vi "PH_AxisGUI_BaseClass.panel.vi"(0 "object ref":refnum<vi>, 5 "error in (no error)":errorcluster) -> (19 "error out":errorcluster)   [LabVIEW 2014, in "PH_AxisGUI_BaseClass.lvlib"]
doc: "License Agreement for this software:\n\nCopyright (C)\nGesellschaft für Schwerionenforschung, GSI\nPlanckstr. 1\n64291 Darmstadt\nGermany\n\nContact: D.Beck@gsi.de \n\nThis program is free software; you can redistribute it and/or modify it under the terms of the GNU General Public License as published by the Free Software Foundation; either version 2 of the license, or (at your option) any later version.\n\nThis program is distributed in the hope that it will be useful, but WITHOUT ANYW ARRANTY; without even the implied warranty of MERCHANTABILITY or FITNESS FOR A PARTICULAR PURPOSE. See the GNU General License for more details (http://www.gnu.org).\n\nGesellschaft für Schwerionenforschung, GSI\nPlanckstr. 1, 64291 Darmstadt, Germany\nFor all questions and ideas contact: M.Richter@gsi.de, H.Brand@gsi.de or D.Beck@gsi.de.\nLast update: 18-DEC-2002"
uses:
  PH_AxisGUI_BaseClass.lvlib
  PH_Stepmotor_BaseClass/PH_Stepmotor_BaseClass.Axis Settings.ctl
  PH_Stepmotor_BaseClass/PH_Stepmotor_BaseClass.Motor Type.ctl
  PH_Stepmotor_BaseClass/PH_Stepmotor_BaseClass.Axis Address.ctl
  PH_Stepmotor_BaseClass/PH_Stepmotor_BaseClass.Axis Activity.ctl
  PH_AxisGUI_BaseClass.Axis GUI Refs.ctl
  PH_Stepmotor_BaseClass/PH_Stepmotor_BaseClass.Axis Direction.ctl
  PH_Common/PH_Common.lvlib
  PH_Stepmotor_BaseClass/PH_Stepmotor_BaseClass.lvlib
  PH_Class/PH_Class.lvlib
panel:
  out "Activity":T1
  out "Status Bar":u32(colorbox)=16777088 caption="Axis1"
  out "Status":u32(colorbox)=6618880 caption="Axis1"
  in  "Stop":bool caption="SetZero"
  in  "Tab Control":enum32{"Move", "Settings", "Info"}(tab)
  in  "Clear Error":bool
  in  "Forth":bool caption="? Steps"
  in  "Back":bool caption="? Steps"
  in  "Target":string="0" caption="Steps"
  in  "Settings":T2={"Sign change"=FALSE, "Width"=0.0, "Calibration"=0.0, "Unit"="Steps", "Motor Type"=enum."Unspecific", "Unit Width"="", "Unit CF"=""}
  out "Address":T4={"Instance"="N/A", "Motor Nr"=0}
  in  "SetZero":bool
  in  "Reset":bool
  in  "Delete":bool
  # "PCS"
  # "3.40"
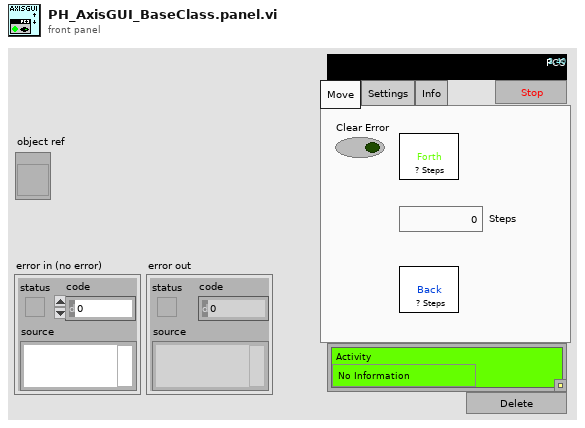
[diagram p1: front panel]
types:
  T1 = typedef "PH_Stepmotor_BaseClass.lvlib/PH_Stepmotor_BaseClass.Axis Activity.ctl" = enum16{"No Information", "stopped", "running", "Failure", "Alarm", "stopped at backward ES", "stopped at foreward ES"}
  T2 = typedef "PH_Stepmotor_BaseClass.lvlib/PH_Stepmotor_BaseClass.Axis Settings.ctl" = cluster{"Sign change":bool, "Width":dbl, "Calibration":dbl, "Unit":string, "Motor Type":T3, "Unit Width":string, "Unit CF":string}
  T3 = typedef "PH_Stepmotor_BaseClass.lvlib/PH_Stepmotor_BaseClass.Motor Type.ctl" = enum16{"Unspecific", "OWIS 49.120.2633", "OWIS 49.060.1033", "OWIS 43.040.2558", "Diamond Motion 2200 series", "OWIS 49.120.266B.MV6", "Calorimeter", "Linear Stage 1", "MICOS VT-80", "MICOS VT-80 S", "Standa Rotstage nt0.95A", "PUF RA 320.200", "PUF RA 800.200", "PUF RA 800.400", "PUF RA 400.50", "1324.nn.800.50", "1324.n9c.800.50", "1324.nn.320.200", "1324.nn.400.200", "1324.nn.800.200", "1324.nn.400.50", "1324.8c9c.800.50", "1324.8c9c.400.200"}
  T4 = typedef "PH_Stepmotor_BaseClass.lvlib/PH_Stepmotor_BaseClass.Axis Address.ctl" = cluster{"Instance":string, "Motor Nr":i32}
  T5 = typedef "PH_AxisGUI_BaseClass.lvlib/PH_AxisGUI_BaseClass.Axis GUI Refs.ctl" = cluster{"Back":refnum<vi>, "Forth":refnum<vi>, "Status":refnum<vi>, "Target":refnum<vi>, "Address":refnum<vi>, "Status Bar":refnum<vi>, "Settings":refnum<vi>, "Activity":refnum<vi>, "Clear Error":refnum<vi>}
  T6 = typedef "PH_Stepmotor_BaseClass.lvlib/PH_Stepmotor_BaseClass.Axis Direction.ctl" = enum16{"forward", "backward"}
  T7 = typedef "PH_AxisGUI_BaseClass.lvlib/PH_AxisGUI_BaseClass.i attribute.ctl" = cluster{"Axes":T8[]}
  T8 = typedef "PH_AxisGUI_BaseClass.lvlib/PH_AxisGUI_BaseClass.Axis Attributes.ctl" = cluster{"Axis GUI Refs":T5, "Address":T4, "Name":string, "Label \"Back\"":string, "Labell \"Forth\"":string, "Moving?":bool}
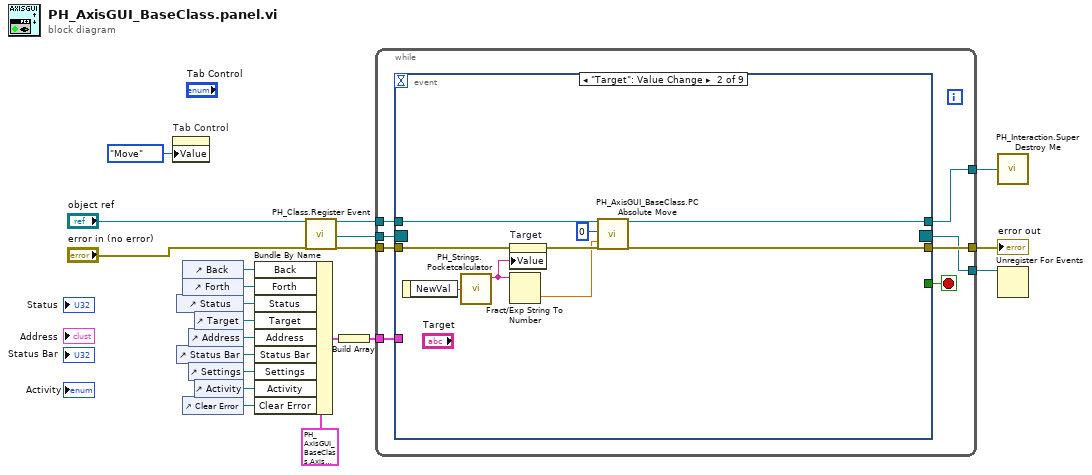
[diagram p0: block diagram]
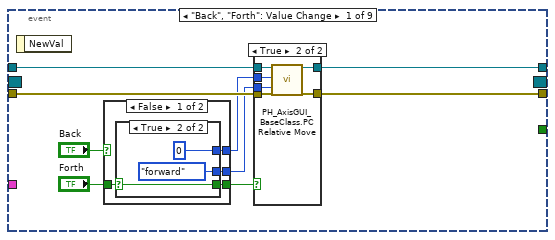
[diagram p2: hidden frame]
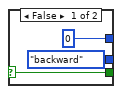
[diagram p3: hidden frame]
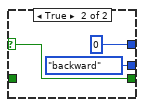
[diagram p4: hidden frame]
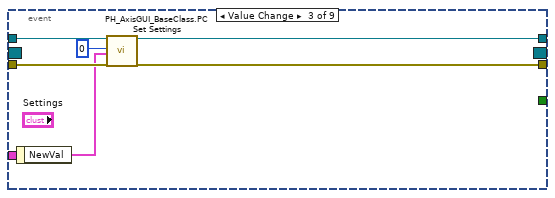
[diagram p6: hidden frame]
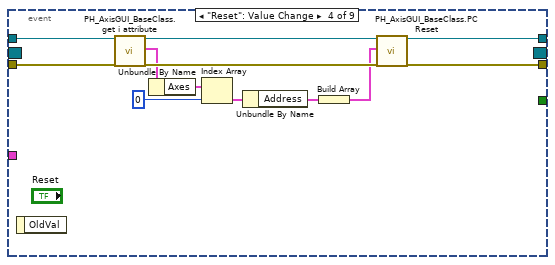
[diagram p7: hidden frame]
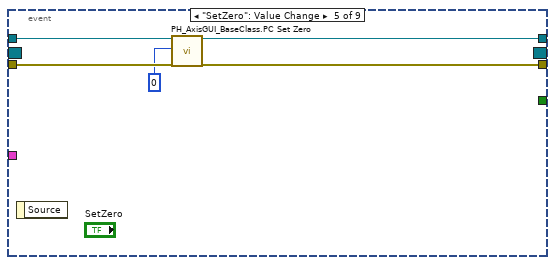
[diagram p8: hidden frame]
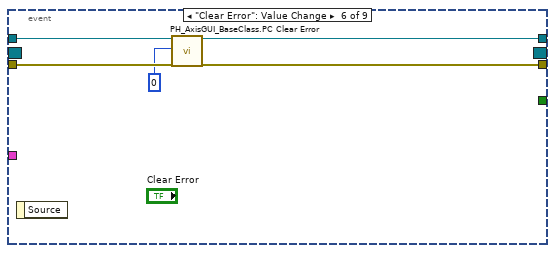
[diagram p9: hidden frame]
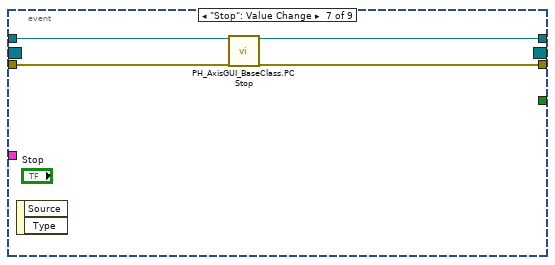
[diagram p10: hidden frame]
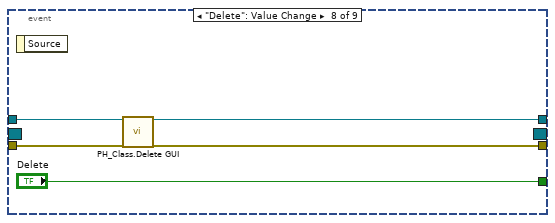
[diagram p11: hidden frame]
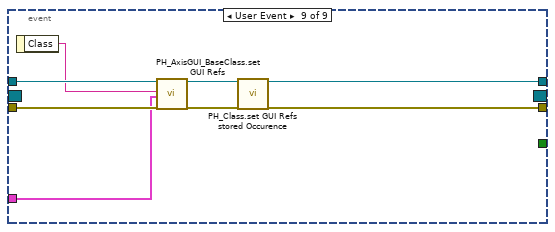
[diagram p12: hidden frame]
diagram:
  n1 = property on="Tab Control" class="TabCtl (strict)"("Value"=enum32{"Move", "Settings", "Info"}."Move" ("Tab Control")) -> ()  [unwired: 2 in, 2 out]
  n2 = control-ref of="Status"() -> (w15:refnum<vi>)
  n3 = control-ref of="Status Bar"() -> (w11:refnum<vi>)
  n4 = control-ref of="Back"() -> (w17:refnum<vi>)
  n5 = control-ref of="Forth"() -> (w16:refnum<vi>)
  n6 = control-ref of="Clear Error"() -> (w8:refnum<vi>)
  n7 = control-ref of="Address"() -> (w12:refnum<vi>)
  n8 = control-ref of="Settings"() -> (w13:refnum<vi>)
  n9 = control-ref of="Target"() -> (w14:refnum<vi>)
  n10 = control-ref of="Activity"() -> (w10:refnum<vi>)
  n11 = Bundle By Name(cluster=T5 {"Back"=refnum, "Forth"=refnum, "Status"=refnum, "Target"=refnum, "Address"=refnum, "Status Bar"=refnum, "Settings"=refnum, "Activity"=refnum, "Clear Error"=refnum} ("GUI Refs"), "Back"=w17, "Forth"=w16, "Status"=w15, "Target"=w14, "Address"=w12, "Status Bar"=w11, "Settings"=w13, "Activity"=w10, "Clear Error"=w8) -> (w18:T5)
  n12 = call "PH_Class.Register Event.vi"("i ref in"="object ref", "error in (no error)"="error in (no error)") -> ("i ref out"=w7:refnum<vi>, "Event Registration Refnum"=w5:refnum<event-registration>, "error out"=w6:errorcluster)  [unwired: 15 in]
  n13 = Build Array(w18) -> (w4:T5[])
  n14 = while {
    tunnel: w7 -> [w26]
    tunnel: [w25] -> w20
    tunnel: w6 -> [w28]
    tunnel: [w27] -> w21
    tunnel: w5 -> [w24]
    tunnel: w4 -> [w23]
    tunnel: [w22] -> w1
    stop <- w29 stop-if-true
    n15 = event shown="[1] \"Target\": Value Change" {
      selector: w24 -> [_ _ _ _ _ _ _ _ _]
      dyn-events: [_ _ _ _ _ _ _ _ _] -> w22
      timeout: _ -> [_ _ _ _ _ _ _ _ _]
      tunnel: [_ _ _ _ _ _ _ "Delete" _] -> w29
      tunnel: w26 -> [w37 w62 w74 w82 w88 w93 w99 w103 w113]
      tunnel: w28 -> [w38 w61 w73 w86 w91 w96 w100 w104 w112]
      tunnel: [w34 w67 w72 w84 w89 w94 w97 w101 w108] -> w27
      tunnel: [w35 w66 w71 w85 w90 w95 w98 w102 w106] -> w25
      tunnel: w23 -> [_ _ _ _ _ _ _ _ w109]
      event "Back", "Forth": Value Change {
        n16 = event-data() -> ()  [unwired: 1 in, 1 out]
        n17 = case shown="False" "Back" {
          selector: "Back" -> [_ w49]
          tunnel: [w42 0] -> w33
          tunnel: [w41 PH_Stepmotor_BaseClass.Axis_Direction."backward" ("direction")] -> w36
          tunnel: "Forth" -> [w40 _]
          tunnel: [w39 w49] -> w30
          frame False {
            n18 = case shown="True" w40 {
              selector: w40 -> [w43 w46]
              tunnel: [0 0] -> w42
              tunnel: [PH_Stepmotor_BaseClass.Axis_Direction."backward" ("direction") PH_Stepmotor_BaseClass.Axis_Direction."forward" ("direction")] -> w41
              tunnel: [w43 w46] -> w39
              frame False {
              }
              frame True {
              }
            }
          }
          frame True {
          }
        }
        n19 = case shown="True" w30 {
          tunnel: w38 -> [w52 w59]
          tunnel: w37 -> [w53 w58]
          tunnel: w36 -> [_ w57]
          tunnel: [w53 w56] -> w35
          tunnel: [w52 w55] -> w34
          tunnel: w33 -> [_ w54]
          frame False {
          }
          frame True {
            n20 = call "PH_AxisGUI_BaseClass.PC Relative Move.vi"("i ref in"=w58, "Axis"=w54, "direction"=w57, "error in"=w59) -> ("i ref out"=w56:refnum<vi>, "error out"=w55:errorcluster)  [unwired: 14 in]
          }
        }
      }
      event "Target": Value Change {
        n21 = event-data() -> ("NewVal"=w68:string)  [unwired: 1 in]
        n22 = call "PH_Strings.Pocketcalculator.vi"("Input"=w68) -> ("String Double"=w65:string)  [unwired: 3 out]
        n23 = property on="Target" class="Str"(error in=w61, "Value"=w65) -> (error out=w64:errorcluster)  [unwired: 1 in, 1 out]
        n24 = Fract/Exp String To Number(string=w65) -> (number=w63:dbl)  [unwired: 3 in, 1 out]
        n25 = call "PH_AxisGUI_BaseClass.PC Absolute Move.vi"("i ref in"=w62, "Axis"=0, "Position [Units]"=w63, "error in"=w64) -> ("i ref out"=w66:refnum<vi>, "error out"=w67:errorcluster)  [unwired: 14 in]
      }
      event Value Change {
        n26 = event-data() -> ("NewVal"=w70:T2)  [unwired: 1 in]
        n27 = call "PH_AxisGUI_BaseClass.PC Set Settings.vi"("VI in"=w74, "Axis"=0 ("index"), "NewVal"=w70, "error in (no error)"=w73) -> ("VI out"=w71:refnum<vi>, "error out"=w72:errorcluster)  [unwired: 14 in]
      }
      event "Reset": Value Change {
        n28 = event-data() -> ()  [unwired: 1 in, 1 out]
        n29 = call "PH_AxisGUI_BaseClass.get i attribute.vi"("i ref in"=w82, "error in (no error)"=w86) -> ("i ref out"=w81:refnum<vi>, "i attribute"=w80:T7, "error out"=w83:errorcluster)  [unwired: 15 in]
        n30 = Unbundle By Name(w80) -> ("Axes"=w79:T8[])
        n31 = Index Array(array=w79, index=0) -> (element=w78:T8)
        n32 = Unbundle By Name(w78) -> ("Address"=w77:T4)
        n33 = Build Array(w77) -> (w76:T4[])
        n34 = call "PH_AxisGUI_BaseClass.PC Reset.vi"("i ref in"=w81, "Addresses"=w76, "error in"=w83) -> ("i ref out"=w85:refnum<vi>, "error out"=w84:errorcluster)  [unwired: 15 in]
      }
      event "SetZero": Value Change {
        n35 = event-data() -> ()  [unwired: 1 in, 1 out]
        n36 = call "PH_AxisGUI_BaseClass.PC Set Zero.vi"("VI in"=w88, "Axis"=0 ("index"), "error in (no error)"=w91) -> ("VI out"=w90:refnum<vi>, "error out"=w89:errorcluster)  [unwired: 15 in]
      }
      event "Clear Error": Value Change {
        n37 = event-data() -> ()  [unwired: 1 in, 1 out]
        n38 = call "PH_AxisGUI_BaseClass.PC Clear Error.vi"("i ref in"=w93, "Axis"=0 ("index"), "error in"=w96) -> ("i ref out"=w95:refnum<vi>, "error out"=w94:errorcluster)  [unwired: 15 in]
      }
      event "Stop": Value Change {
        n39 = event-data() -> ()  [unwired: 1 in, 2 out]
        n40 = call "PH_AxisGUI_BaseClass.PC Stop.vi"("VI in"=w99, "error in (no error)"=w100) -> ("VI out"=w98:refnum<vi>, "error out"=w97:errorcluster)  [unwired: 16 in]
      }
      event "Delete": Value Change {
        n41 = event-data() -> ()  [unwired: 1 in, 1 out]
        n42 = call "PH_Class.Delete GUI.vi"("VI in"=w103, "error in (no error)"=w104) -> ("VI out"=w102:refnum<vi>, "error out"=w101:errorcluster)  [unwired: 16 in]
      }
      event User Event {
        n43 = event-data() -> ("Class"=w110:string)  [unwired: 1 in]
        n44 = call "PH_AxisGUI_BaseClass.set GUI Refs.vi"("i ref in"=w113, "Class"=w110, "Axis GUI Base Class Refs"=w109, "error in"=w112) -> ("i ref out"=w107:refnum<vi>, "error out"=w111:errorcluster)  [unwired: 14 in]
        n45 = call "PH_Class.set GUI Refs stored Occurence.vi"("i ref in"=w107, "error in (no error)"=w111) -> ("i ref out"=w106:refnum<vi>, "error out"=w108:errorcluster)  [unwired: 16 in]
      }
    }
  }
  "error out" <- w21
  n46 = call "PH_Interaction.Super Destroy Me.vi"("i ref out"=w20) -> ()
  n47 = Unregister For Events(event registration refnum=w1) -> ()  [unwired: 1 in, 1 out]
